vi "Initialize.vi"(7 "3D Picture Refnum":refnum<vi>, 8 "error in":errorcluster, 11 "AR Example.lvlib:UI.lvclass":refnum<class "UI.lvclass">) -> (0 "error out":errorcluster, 3 "App out":refnum<class "App.lvclass">)   [LabVIEW 2020, in "AR Example.lvlib" / "App.lvclass"]
uses:
  App.lvclass
  UI/Tab Control.ctl
  UI/UI.lvclass
  g_ar_toolkit.image/New Image (ARGB).vi
  g_ar_toolkit.image/New Image (Greyscale).vi
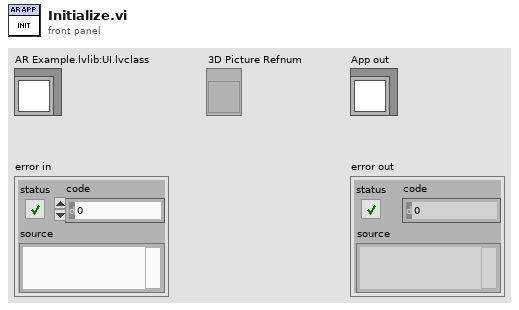
[diagram p1: front panel]
types:
  T1 = typedef "AR Example.lvlib/UI.lvclass/Tab Control.ctl" = enum8{"Config Load", "Camera Selection", "Camera Calibration"}
  T2 = typedef "g_ar_toolkit.image.lvlib/ARGB Image.ctl" = refnum<data-value>
  T3 = typedef "g_ar_toolkit.image.lvlib/Greyscale Image.ctl" = refnum<data-value>
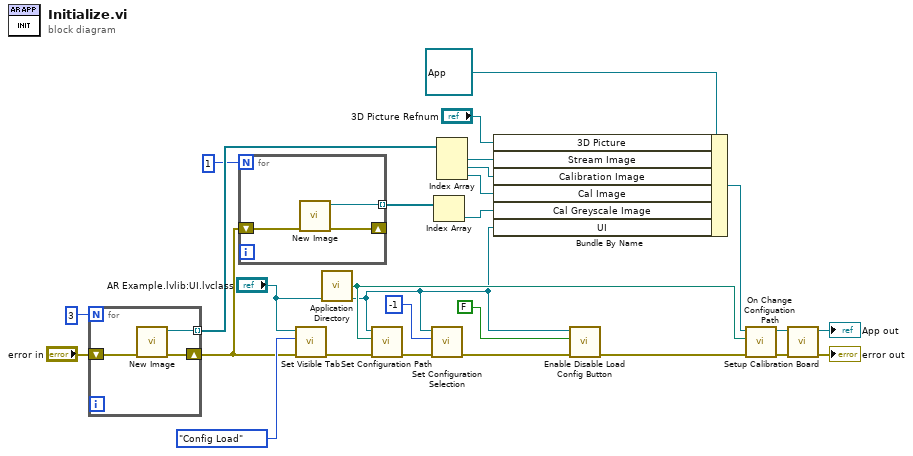
[diagram p0: block diagram]
diagram:
  n1 = for {
    N: 3 -> [_]
    tunnel: [w28] -> w11 mode=indexing
    shift-right: [w29] -> w4
    shift-left: "error in" -> [w27]
    n2 = call-poly "New Image.vi"("error in (no error)"=w27) -> ("error out"=w29:errorcluster, "New ARGB Image"=w28:T2)  [unwired: 9 in]
  }
  n3 = for {
    N: 1 -> [_]
    shift-right: [w31] -> _
    shift-left: w4 -> [w32]
    tunnel: [w30] -> w2 mode=indexing
    n4 = call-poly "New Image.vi"("error in (no error)"=w32) -> ("error out"=w31:errorcluster, "New Greyscale Image"=w30:T3)  [unwired: 9 in]
  }
  n5 = call-dynamic "Set Visible Tab.vi"("error in (no error)"=w4, "Value"=Tab_Control."Config Load", "UI in"="AR Example.lvlib:UI.lvclass") -> ("error out"=w19:errorcluster)  [unwired: 8 in]
  n6 = call <vilib>:"Application Directory.vi"() -> ("Application Directory"=w17:path)
  n7 = call-dynamic "Set Configuration Path.vi"("error in (no error)"=w19, "Value"=w17, "UI in"="AR Example.lvlib:UI.lvclass") -> ("error out"=w25:errorcluster)  [unwired: 8 in]
  n8 = call-dynamic "Set Configuration Selection.vi"("error in (no error)"=w25, "Selection"=-1, "UI in"="AR Example.lvlib:UI.lvclass") -> ("error out"=w23:errorcluster)  [unwired: 8 in]
  n9 = Index Array(array=w2) -> (element=w1:T3)  [unwired: 1 in]
  n10 = Index Array(array=w11) -> (element #1=w12:T2, element #2=w10:T2, element #3=w5:T2)  [unwired: 3 in]
  n11 = Bundle By Name(cluster=refnum<class "App.lvclass"> refnum ("App out"), "3D Picture"="3D Picture Refnum", "Stream Image"=w12, "Calibration Image"=w10, "Cal Image"=w5, "Cal Greyscale Image"=w1, "UI"="AR Example.lvlib:UI.lvclass") -> (w22:refnum<class "App.lvclass">)
  n12 = call-dynamic "Enable Disable Load Config Button.vi"("error in (no error)"=w23, "Enable?"=FALSE, "UI in"="AR Example.lvlib:UI.lvclass") -> ("error out"=w21:errorcluster)  [unwired: 8 in]
  n13 = call "On Change Configuation Path.vi"("error in (no error)"=w21, "Path"=w17, "App in"=w22) -> ("error out"=w9:errorcluster, "App out"=w7:refnum<class "App.lvclass">)  [unwired: 7 in]
  n14 = call "Setup Calibration Board.vi"("error in (no error)"=w9, "App in"=w7) -> ("error out"=→"error out":errorcluster, "App out"=→"App out":refnum<class "App.lvclass">)  [unwired: 8 in]
